vi "sendValue.vi"(8 "error in (no error)":errorcluster, 10 "data":variant, 11 "detailedState in":refnum<class "detailedState.lvclass">) -> (0 "error out":errorcluster, 2 "function return":i32, 3 "detailedState out":refnum<class "detailedState.lvclass">)   [LabVIEW 2016, in "SALLV_EXA_Messaging.lvlib" / "detailedState.lvclass"]
uses:
  detailedState.lvclass
  ts_sallv_MtAtElectrometer/DataTypes/logevent_detailedState.ctl
  detailedState.lvclass/detailedState.ctl
  ts_sallv_MtAtElectrometer/SALLV_MtAtElectrometer.lvlib
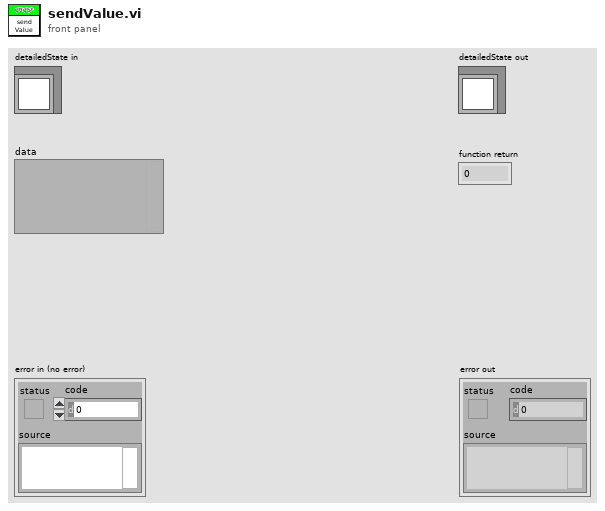
[diagram p1: front panel]
types:
  T1 = typedef "SALLV_MtAtElectrometer.lvlib/logevent_detailedState.ctl" = cluster{"detailedState":i32, "priority":i32}
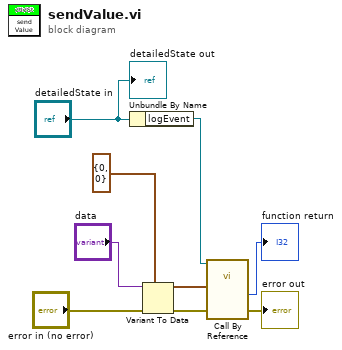
[diagram p0: block diagram]
diagram:
  n1 = Unbundle By Name("detailedState in") -> ("logEvent"=w6:refnum<vi>)
  n2 = Variant To Data(error in="error in (no error)", type=T1 {"detailedState"=0, "priority"=0} ("logevent_detailedState_Ctl"), Variant="data") -> (data=w4:T1, error out=w3:errorcluster)
  n3 = call-by-ref "?"(reference=w6, "error in (no error)"=w3, "logevent_detailedState_Ctl"=w4) -> ("error out"=→"error out":errorcluster, "function return"=→"function return":i32)  [unwired: 8 in, 3 out]
  "detailedState out" <- "detailedState in"
